vi "DSF.Engine.Execution.Builder.Parse.vi"(6 "Data Type Buffers in":T1, 8 "error in (no error)":errorcluster, 9 "Transfer ID":i32, 10 "Plugin ID":i32, 11 "Builder in":refnum<class "DSF.Engine.Execution.Builder.lvclass">) -> (0 "error out":errorcluster, 3 "Builder out":refnum<class "DSF.Engine.Execution.Builder.lvclass">, 4 "Data Type Buffers out":T1)   [LabVIEW 2016, in "DSF.Engine.lvlib" / "DSF.Engine.Execution.Builder.lvclass"]
uses:
  DSF.Engine.Execution.Builder.lvclass
  DSF.Engine.Execution.Builder.Type Buffers.ctl
  Cache/DSF.Engine.Memory.Cache.Framework.lvclass
  Cache/DSF.Engine.Memory.Cache.Plugin.lvclass
  Pointer/DSF.Engine.Memory.Pointer.VS Channels.lvclass
  Buffer/DSF.Engine.Memory.Buffer.lvclass
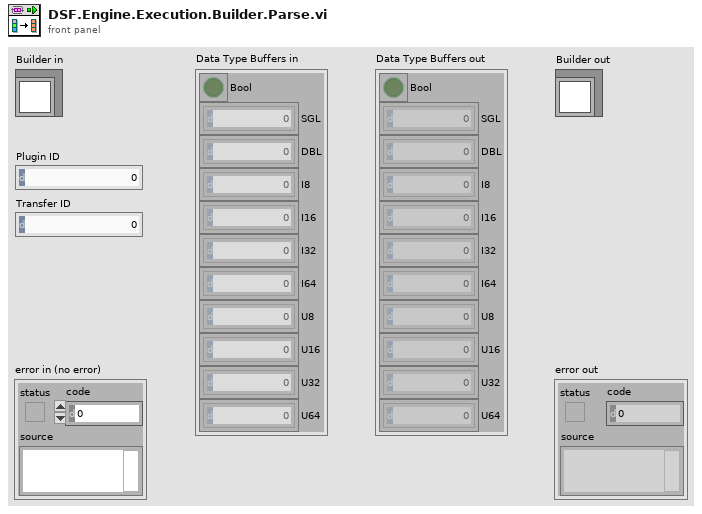
[diagram p1: front panel]
types:
  T1 = typedef "DSF.Engine.lvlib/DSF.Engine.Execution.Builder.lvclass/DSF.Engine.Execution.Builder.Type Buffers.ctl" = cluster{"Bool":bool[], "SGL":sgl[], "DBL":dbl[], "I8":i8[], "I16":i16[], "I32":i32[], "I64":i64[], "U8":u8[], "U16":u16[], "U32":u32[], "U64":u64[]}
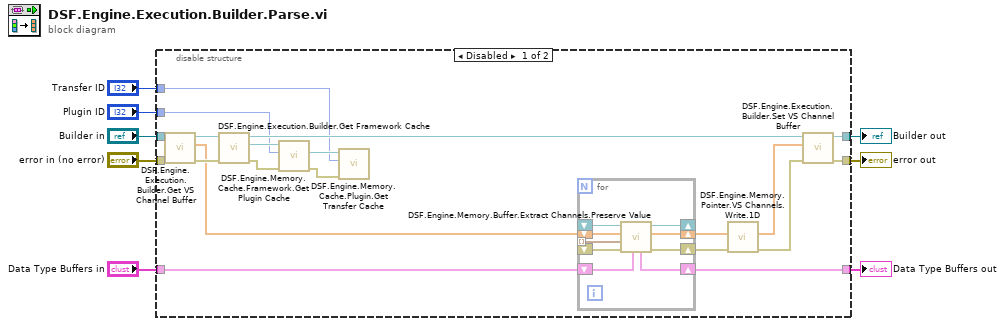
[diagram p0: block diagram]
diagram:
  n1 = disable-structure shown="Disabled" {
    disable-tunnel: "Builder in" -> [w26 w43]
    disable-tunnel: "error in (no error)" -> [w25 _]
    disable-tunnel: [w24 w43] -> w6
    disable-tunnel: [w23 _] -> w5
    disable-tunnel: "Plugin ID" -> [w22 _]
    disable-tunnel: "Transfer ID" -> [w21 _]
    disable-tunnel: "Data Type Buffers in" -> [w14 _]
    disable-tunnel: [w13 _] -> w1
    frame Disabled {
      n2 = call "DSF.Engine.Execution.Builder.Get VS Channel Buffer.vi"("error in (no error)"=w25, "Builder in"=w26) -> ("error out"=w28:errorcluster, "VS Channel Buffer"=w20:dbl[], "Builder out"=w29:refnum<class "DSF.Engine.Execution.Builder.lvclass">)  [unwired: 7 in]
      n3 = call "DSF.Engine.Execution.Builder.Get Framework Cache.vi"("error in (no error)"=w28, "Builder in"=w29) -> ("error out"=w30:errorcluster, "Framework Cache"=w33:refnum<class "DSF.Engine.Memory.Cache.Framework.lvclass">, "Builder out"=w27:refnum<class "DSF.Engine.Execution.Builder.lvclass">)  [unwired: 7 in]
      n4 = call "DSF.Engine.Memory.Cache.Framework.Get Plugin Cache.vi"("error in (no error)"=w30, "Plugin ID"=w22, "Framework Cache in"=w33) -> ("error out"=w31:errorcluster, "Plugin Cache"=w32:refnum<class "DSF.Engine.Memory.Cache.Plugin.lvclass">)  [unwired: 6 in, 1 out]
      n5 = call "DSF.Engine.Memory.Cache.Plugin.Get Transfer Cache.vi"("error in (no error)"=w31, "Transfer ID"=w21, "Plugin Cache in"=w32) -> ("Transfer Cache"=w12:refnum<class "DSF.Engine.Memory.Cache.Transfer.lvclass">)  [unwired: 6 in, 2 out]
      n6 = for {
        tunnel: [w37] -> w11 mode=indexing
        shift-right: [w40] -> w18
        shift-left: w20 -> [w41]
        shift-right: [w39] -> w19
        shift-left: [w42] -> w17
        shift-right: [w35] -> w13
        shift-left: w14 -> [w36]
        shift-right: [w34] -> _
        shift-left: [w38] -> w10
        n7 = call "DSF.Engine.Memory.Buffer.Extract Channels.Preserve Value.vi"("Data Type Buffers in"=w36, "error in (no error)"=w42, "Channel Configuration"=w37, "VS Channels Array in"=w41, "Buffer in"=w38) -> ("error out"=w39:errorcluster, "VS Channels Array out"=w40:dbl[], "Buffer out"=w34:refnum<class "DSF.Engine.Memory.Buffer.lvclass">, "Data Type Buffers out"=w35:T1)  [unwired: 3 in]
      }
      n8 = call "DSF.Engine.Memory.Pointer.VS Channels.Write.1D.vi"("error in (no error)"=w19, "Channels Array in"=w18) -> ("error out"=w16:errorcluster, "Channels Array out"=w15:dbl[], "VS Channels Pointer in"=w9:refnum<class "DSF.Engine.Memory.Pointer.VS Channels.lvclass">)  [unwired: 5 in, 2 out]
      n9 = call "DSF.Engine.Execution.Builder.Set VS Channel Buffer.vi"("error in (no error)"=w16, "VS Channel Buffer"=w15, "Builder in"=w27) -> ("error out"=w23:errorcluster, "Builder out"=w24:refnum<class "DSF.Engine.Execution.Builder.lvclass">)  [unwired: 7 in]
    }
    frame Enabled {
    }
  }
  "error out" <- w5
  "Builder out" <- w6
  "Data Type Buffers out" <- w1
